vi "CAN 6 SPARK MAX Drivetrain Config.vi"() -> (14 "SPARK MAX Ref":T1={"FrontLeftMaster"={"DeviceStatus"={"status"=FALSE, "code"=0, "source"=""}, "Type"=enum."PWM", "PWM"={"PWM Channel"=enum."PWM 1", "DeadBand"={"Name"="", "maxPositivePwm"=0, "minPositivePwm"=0, "centerPwm"=0, "maxNegativePwm"=0, "minNegativePwm"=0, "angularRange"=0}}, "CAN"={"Device Number"=0, "SetOutput VI Ref"=variant(enum8{"Percent VBus", "Current", "Speed", "Position", "Voltage"} enum."Percent VBus"), "GetOutput VI Ref"=variant(refnum<k1> refnum), "Enable VI Ref"=variant(dbl 12.0), "Disable VI Ref"=variant(enum8{"Percent VBus", "Speed", "Position", "Slave", "Unchanged / Invalid", "Voltage Compensation", "Current", "Motion Profile"} enum."Percent VBus"), "Data"=variant}, "Invert"=FALSE, "DIO PWM"={"PWM \"Enable\" Channel"=enum."Invalid", "DIOChannel"=enum."Invalid", "PWM Rate"=0.0}}, "FrontLeftSlave1"={"DeviceStatus"={"status"=FALSE, "code"=0, "source"=""}, "Type"=enum."PWM", "PWM"={"PWM Channel"=enum."PWM 1", "DeadBand"={"Name"="", "maxPositivePwm"=0, "minPositivePwm"=0, "centerPwm"=0, "maxNegativePwm"=0, "minNegativePwm"=0, "angularRange"=0}}, "CAN"={"Device Number"=0, "SetOutput VI Ref"=variant(enum8{"Percent VBus", "Current", "Speed", "Position", "Voltage"} enum."Percent VBus"), "GetOutput VI Ref"=variant(refnum<k1> refnum), "Enable VI Ref"=variant(dbl 12.0), "Disable VI Ref"=variant(enum8{"Percent VBus", "Speed", "Position", "Slave", "Unchanged / Invalid", "Voltage Compensation", "Current", "Motion Profile"} enum."Percent VBus"), "Data"=variant}, "Invert"=FALSE, "DIO PWM"={"PWM \"Enable\" Channel"=enum."Invalid", "DIOChannel"=enum."Invalid", "PWM Rate"=0.0}}, "FrontLeftSlave2"={"DeviceStatus"={"status"=FALSE, "code"=0, "source"=""}, "Type"=enum."PWM", "PWM"={"PWM Channel"=enum."PWM 1", "DeadBand"={"Name"="", "maxPositivePwm"=0, "minPositivePwm"=0, "centerPwm"=0, "maxNegativePwm"=0, "minNegativePwm"=0, "angularRange"=0}}, "CAN"={"Device Number"=0, "SetOutput VI Ref"=variant(enum8{"Percent VBus", "Current", "Speed", "Position", "Voltage"} enum."Percent VBus"), "GetOutput VI Ref"=variant(refnum<k1> refnum), "Enable VI Ref"=variant(dbl 12.0), "Disable VI Ref"=variant(enum8{"Percent VBus", "Speed", "Position", "Slave", "Unchanged / Invalid", "Voltage Compensation", "Current", "Motion Profile"} enum."Percent VBus"), "Data"=variant}, "Invert"=FALSE, "DIO PWM"={"PWM \"Enable\" Channel"=enum."Invalid", "DIOChannel"=enum."Invalid", "PWM Rate"=0.0}}, "FrontRightMaster"={"DeviceStatus"={"status"=FALSE, "code"=0, "source"=""}, "Type"=enum."PWM", "PWM"={"PWM Channel"=enum."PWM 1", "DeadBand"={"Name"="", "maxPositivePwm"=0, "minPositivePwm"=0, "centerPwm"=0, "maxNegativePwm"=0, "minNegativePwm"=0, "angularRange"=0}}, "CAN"={"Device Number"=0, "SetOutput VI Ref"=variant(enum8{"Percent VBus", "Current", "Speed", "Position", "Voltage"} enum."Percent VBus"), "GetOutput VI Ref"=variant(refnum<k1> refnum), "Enable VI Ref"=variant(dbl 12.0), "Disable VI Ref"=variant(enum8{"Percent VBus", "Speed", "Position", "Slave", "Unchanged / Invalid", "Voltage Compensation", "Current", "Motion Profile"} enum."Percent VBus"), "Data"=variant}, "Invert"=FALSE, "DIO PWM"={"PWM \"Enable\" Channel"=enum."Invalid", "DIOChannel"=enum."Invalid", "PWM Rate"=0.0}}, "FrontRightSlave1"={"DeviceStatus"={"status"=FALSE, "code"=0, "source"=""}, "Type"=enum."PWM", "PWM"={"PWM Channel"=enum."PWM 1", "DeadBand"={"Name"="", "maxPositivePwm"=0, "minPositivePwm"=0, "centerPwm"=0, "maxNegativePwm"=0, "minNegativePwm"=0, "angularRange"=0}}, "CAN"={"Device Number"=0, "SetOutput VI Ref"=variant(enum8{"Percent VBus", "Current", "Speed", "Position", "Voltage"} enum."Percent VBus"), "GetOutput VI Ref"=variant(refnum<k1> refnum), "Enable VI Ref"=variant(dbl 12.0), "Disable VI Ref"=variant(enum8{"Percent VBus", "Speed", "Position", "Slave", "Unchanged / Invalid", "Voltage Compensation", "Current", "Motion Profile"} enum."Percent VBus"), "Data"=variant}, "Invert"=FALSE, "DIO PWM"={"PWM \"Enable\" Channel"=enum."Invalid", "DIOChannel"=enum."Invalid", "PWM Rate"=0.0}}, "FrontRightSlave2"={"DeviceStatus"={"status"=FALSE, "code"=0, "source"=""}, "Type"=enum."PWM", "PWM"={"PWM Channel"=enum."PWM 1", "DeadBand"={"Name"="", "maxPositivePwm"=0, "minPositivePwm"=0, "centerPwm"=0, "maxNegativePwm"=0, "minNegativePwm"=0, "angularRange"=0}}, "CAN"={"Device Number"=0, "SetOutput VI Ref"=variant(enum8{"Percent VBus", "Current", "Speed", "Position", "Voltage"} enum."Percent VBus"), "GetOutput VI Ref"=variant(refnum<k1> refnum), "Enable VI Ref"=variant(dbl 12.0), "Disable VI Ref"=variant(enum8{"Percent VBus", "Speed", "Position", "Slave", "Unchanged / Invalid", "Voltage Compensation", "Current", "Motion Profile"} enum."Percent VBus"), "Data"=variant}, "Invert"=FALSE, "DIO PWM"={"PWM \"Enable\" Channel"=enum."Invalid", "DIOChannel"=enum."Invalid", "PWM Rate"=0.0}}})   [LabVIEW 2018]
uses:
  SPARKMAX6Motor.ctl
  <vilib>/Rock Robotics/WPI/MotorControl/WPI_MotorControlDeviceRef.ctl
  <vilib>/Rock Robotics/WPI/MotorControl/WPI_MotorControlType.ctl
  <vilib>/Rock Robotics/SystemInterfaces/DIO/FPGA_DIOPWMChannel.ctl
  <vilib>/Rock Robotics/WPI/PWM/WPI_PWMDeadband.ctl
  <vilib>/Rock Robotics/SystemInterfaces/DIO/FPGA_DIOChannel.ctl
  <vilib>/Rock Robotics/WPI/ThirdParty/REV Robotics/SPARK MAX/Typedef/Spark MAX Status Frames.ctl
  <vilib>/Rock Robotics/WPI/ThirdParty/REV Robotics/SPARK MAX/Typedef/Spark MAX Idle Mode.ctl
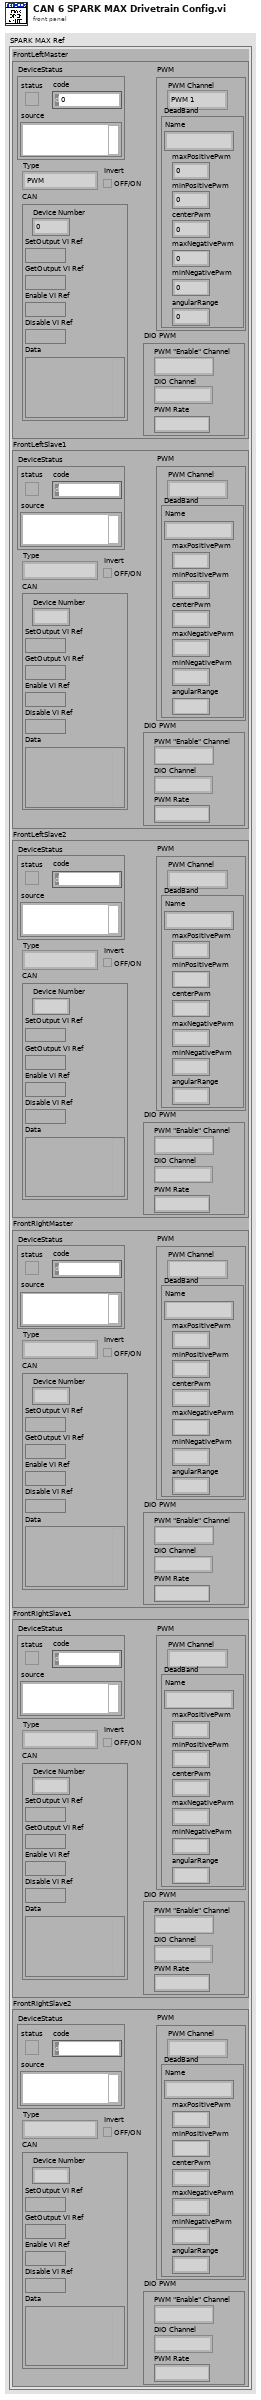
[diagram p1: front panel]
types:
  T1 = typedef "SPARKMAX6Motor.ctl" = cluster{"FrontLeftMaster":T2, "FrontLeftSlave1":T2, "FrontLeftSlave2":T2, "FrontRightMaster":T2, "FrontRightSlave1":T2, "FrontRightSlave2":T2}
  T2 = typedef "WPI_MotorControlDeviceRef.ctl" = cluster{"DeviceStatus":errorcluster, "Type":T3, "PWM":cluster{"PWM Channel":T4, "DeadBand":T5}, "CAN":cluster{"Device Number":u8, "SetOutput VI Ref":variant, "GetOutput VI Ref":variant, "Enable VI Ref":variant, "Disable VI Ref":variant, "Data":variant}, "Invert":bool, "DIO PWM":cluster{"PWM \"Enable\" Channel":T4, "DIOChannel":T6, "PWM Rate":dbl}}
  T3 = typedef "WPI_MotorControlType.ctl" = enum16{"PWM", "CAN", "DIO PWM"}
  T4 = typedef "FPGA_DIOPWMChannel.ctl" = enum8{"PWM 0", "PWM 1", "PWM 2", "PWM 3", "PWM 4", "PWM 5", "PWM 6", "PWM 7", "PWM 8", "PWM 9", "PWM MXP 0", "PWM MXP 1", "PWM MXP 2", "PWM MXP 3", "PWM MXP 4", "PWM MXP 5", "PWM MXP 6", "PWM MXP 7", "PWM MXP 8", "PWM MXP 9", "Invalid"}
  T5 = typedef "WPI_PWMDeadband.ctl" = cluster{"Name":string, "maxPositivePwm":i32, "minPositivePwm":i32, "centerPwm":i32, "maxNegativePwm":i32, "minNegativePwm":i32, "angularRange":u16}
  T6 = typedef "FPGA_DIOChannel.ctl" = enum8{"DIO 0", "DIO 1", "DIO 2", "DIO 3", "DIO 4", "DIO 5", "DIO 6", "DIO 7", "DIO 8", "DIO 9", "DIO MXP 0", "DIO MXP 1", "DIO MXP 2", "DIO MXP 3", "DIO MXP 4", "DIO MXP 5", "DIO MXP 6", "DIO MXP 7", "DIO MXP 8", "DIO MXP 9", "DIO MXP 10", "DIO MXP 11", "DIO MXP 12", "DIO MXP 13", "DIO MXP 14", "DIO MXP 15", "SPI Port CS1", "SPI Port CS2", "SPI Port CS3", "SPI Port MISO", "SPI Port MOSI", "Invalid"}
  T7 = typedef "Spark MAX Idle Mode.ctl" = enum16{"Coast", "Brake"}
  T8 = typedef "Spark MAX Status Frames.ctl" = enum16{"Status 0", "Status 1", "Status 2"}
  T9 = cluster{"P Gain":dbl, "I Gain":dbl, "D Gain":dbl, "F Gain":dbl, "I Zone":dbl, "Min Output":dbl, "Max Output":dbl}
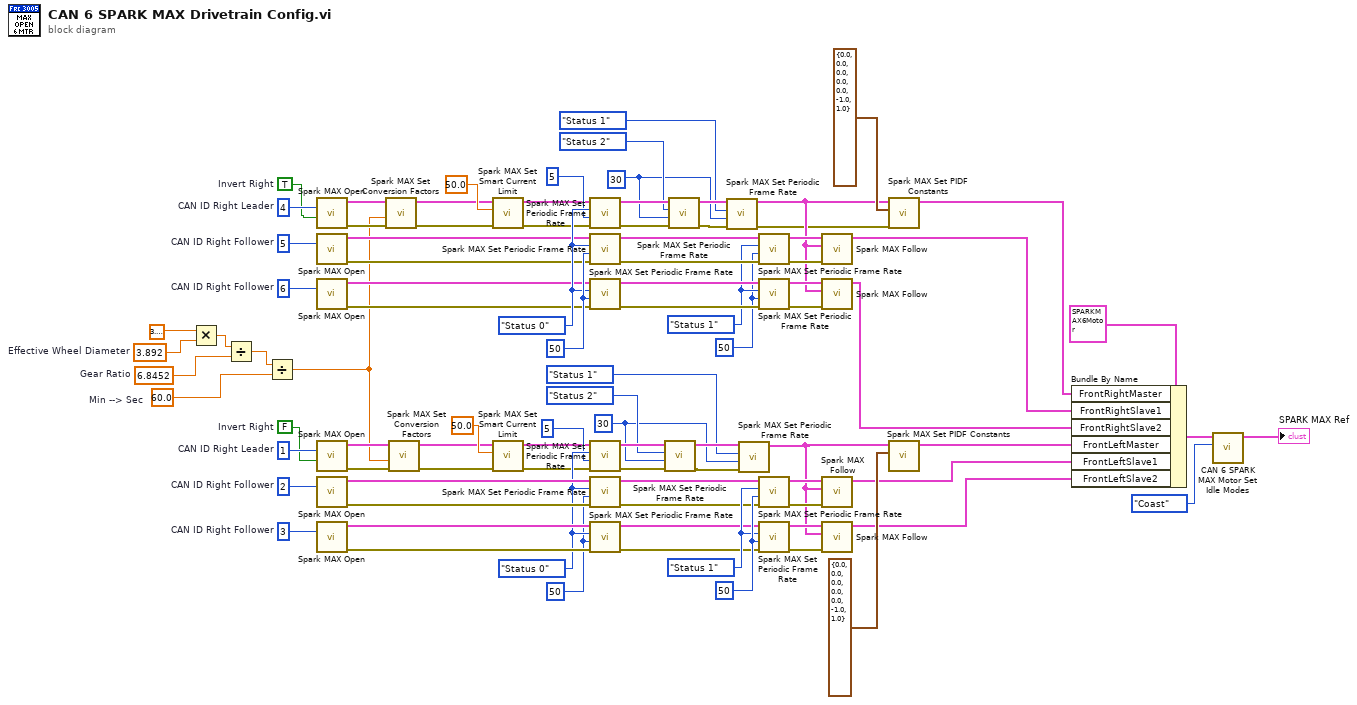
[diagram p0: block diagram]
diagram:
  w1 = 3.892  # Effective Wheel Diameter
  w2 = 6.8452  # Gear Ratio
  w3 = 60.0  # Min --> Sec
  w61 = u16 50 ("Frame rate (ms)")
  w62 = Spark_MAX_Status_Frames."Status 1" ("Frame")
  w60 = u16 50 ("Frame rate (ms)")
  w26 = u16 30 ("Frame rate (ms)")
  w59 = Spark_MAX_Status_Frames."Status 0" ("Frame")
  w54 = u8 6  # CAN ID Right Follower
  w28 = TRUE  # Invert Right
  w52 = u8 4  # CAN ID Right Leader
  w53 = u8 5  # CAN ID Right Follower
  w82 = u16 50 ("Frame rate (ms)")
  w81 = Spark_MAX_Status_Frames."Status 1" ("Frame")
  w83 = u16 50 ("Frame rate (ms)")
  w29 = u16 30 ("Frame rate (ms)")
  w84 = Spark_MAX_Status_Frames."Status 0" ("Frame")
  w90 = u8 3  # CAN ID Right Follower
  w27 = FALSE  # Invert Right
  w92 = u8 1  # CAN ID Right Leader
  w91 = u8 2  # CAN ID Right Follower
  n1 = Multiply(x=3.141592653589793, y=w1) -> (x*y=w5:dbl)
  n2 = Divide(x=w5, y=w2) -> (x/y=w6:dbl)
  n3 = Divide(x=w6, y=w3) -> (x/y=w4:dbl)
  n4 = call <vilib>:"Spark MAX Open.vi"("Invert"=w28, "Device Number"=w52) -> ("error out"=w14:errorcluster, "MotorControlDeviceRef"=w12:T2)  [unwired: 8 in]
  n5 = call <vilib>:"Spark MAX Open.vi"("Device Number"=w53) -> ("error out"=w57:errorcluster, "MotorControlDeviceRef"=w58:T2)  [unwired: 9 in]
  n6 = call <vilib>:"Spark MAX Open.vi"("Device Number"=w54) -> ("error out"=w55:errorcluster, "MotorControlDeviceRef"=w56:T2)  [unwired: 9 in]
  n7 = call <vilib>:"Spark MAX Open.vi"("Invert"=w27, "Device Number"=w92) -> ("error out"=w85:errorcluster, "MotorControlDeviceRef"=w9:T2)  [unwired: 8 in]
  n8 = call <vilib>:"Spark MAX Open.vi"("Device Number"=w91) -> ("error out"=w87:errorcluster, "MotorControlDeviceRef"=w86:T2)  [unwired: 9 in]
  n9 = call <vilib>:"Spark MAX Open.vi"("Device Number"=w90) -> ("error out"=w89:errorcluster, "MotorControlDeviceRef"=w88:T2)  [unwired: 9 in]
  n10 = call <vilib>:"Spark MAX Set Conversion Factors.vi"("error in (no error)"=w14, "Velocity Factor (1)"=w4, "MotorControlDeviceRef in"=w12) -> ("error out"=w13:errorcluster, "MotorControlDeviceRef out"=w11:T2)  [unwired: 7 in]
  n11 = call <vilib>:"Spark MAX Set Conversion Factors.vi"("error in (no error)"=w85, "Velocity Factor (1)"=w4, "MotorControlDeviceRef in"=w9) -> ("error out"=w10:errorcluster, "MotorControlDeviceRef out"=w8:T2)  [unwired: 7 in]
  n12 = call <vilib>:"Spark MAX Set Smart Current Limit.vi"("error in (no error)"=w13, "Primay Current Limit (80A)"=50.0, "MotorControlDeviceRef in"=w11) -> ("error out"=w20:errorcluster, "MotorControlDeviceRef out"=w19:T2)  [unwired: 7 in]
  n13 = call <vilib>:"Spark MAX Set Smart Current Limit.vi"("error in (no error)"=w10, "Primay Current Limit (80A)"=50.0, "MotorControlDeviceRef in"=w8) -> ("error out"=w18:errorcluster, "MotorControlDeviceRef out"=w17:T2)  [unwired: 7 in]
  n14 = call <vilib>:"Spark MAX Set Periodic Frame Rate.vi"("error in"=w20, "Frame rate (ms)"=u16 5, "Frame"=w59, "MotorControlDeviceRef"=w19) -> ("error out"=w44:errorcluster, "MotorControlDeviceRef"=w43:T2)  [unwired: 6 in]
  n15 = call <vilib>:"Spark MAX Set Periodic Frame Rate.vi"("error in"=w57, "Frame rate (ms)"=w60, "Frame"=w59, "MotorControlDeviceRef"=w58) -> ("error out"=w66:errorcluster, "MotorControlDeviceRef"=w63:T2)  [unwired: 6 in]
  n16 = call <vilib>:"Spark MAX Set Periodic Frame Rate.vi"("error in"=w55, "Frame rate (ms)"=w60, "Frame"=w59, "MotorControlDeviceRef"=w56) -> ("error out"=w65:errorcluster, "MotorControlDeviceRef"=w64:T2)  [unwired: 6 in]
  n17 = call <vilib>:"Spark MAX Set Periodic Frame Rate.vi"("error in"=w18, "Frame rate (ms)"=u16 5, "Frame"=w84, "MotorControlDeviceRef"=w17) -> ("error out"=w33:errorcluster, "MotorControlDeviceRef"=w34:T2)  [unwired: 6 in]
  n18 = call <vilib>:"Spark MAX Set Periodic Frame Rate.vi"("error in"=w87, "Frame rate (ms)"=w83, "Frame"=w84, "MotorControlDeviceRef"=w86) -> ("error out"=w77:errorcluster, "MotorControlDeviceRef"=w80:T2)  [unwired: 6 in]
  n19 = call <vilib>:"Spark MAX Set Periodic Frame Rate.vi"("error in"=w89, "Frame rate (ms)"=w83, "Frame"=w84, "MotorControlDeviceRef"=w88) -> ("error out"=w78:errorcluster, "MotorControlDeviceRef"=w79:T2)  [unwired: 6 in]
  n20 = call <vilib>:"Spark MAX Set Periodic Frame Rate.vi"("error in"=w33, "Frame rate (ms)"=w29, "Frame"=Spark_MAX_Status_Frames."Status 2", "MotorControlDeviceRef"=w34) -> ("error out"=w36:errorcluster, "MotorControlDeviceRef"=w35:T2)  [unwired: 6 in]
  n21 = call <vilib>:"Spark MAX Set Periodic Frame Rate.vi"("error in"=w44, "Frame rate (ms)"=w26, "Frame"=Spark_MAX_Status_Frames."Status 2", "MotorControlDeviceRef"=w43) -> ("error out"=w41:errorcluster, "MotorControlDeviceRef"=w42:T2)  [unwired: 6 in]
  n22 = call <vilib>:"Spark MAX Set Periodic Frame Rate.vi"("error in"=w41, "Frame rate (ms)"=w26, "Frame"=Spark_MAX_Status_Frames."Status 1", "MotorControlDeviceRef"=w42) -> ("error out"=w37:errorcluster, "MotorControlDeviceRef"=w38:T2)  [unwired: 6 in]
  n23 = call <vilib>:"Spark MAX Set Periodic Frame Rate.vi"("error in"=w36, "Frame rate (ms)"=w29, "Frame"=Spark_MAX_Status_Frames."Status 1", "MotorControlDeviceRef"=w35) -> ("MotorControlDeviceRef"=w32:T2)  [unwired: 6 in, 1 out]
  n24 = call <vilib>:"Spark MAX Set Periodic Frame Rate.vi"("error in"=w66, "Frame rate (ms)"=w61, "Frame"=w62, "MotorControlDeviceRef"=w63) -> ("error out"=w68:errorcluster, "MotorControlDeviceRef"=w67:T2)  [unwired: 6 in]
  n25 = call <vilib>:"Spark MAX Set Periodic Frame Rate.vi"("error in"=w65, "Frame rate (ms)"=w61, "Frame"=w62, "MotorControlDeviceRef"=w64) -> ("error out"=w69:errorcluster, "MotorControlDeviceRef"=w70:T2)  [unwired: 6 in]
  n26 = call <vilib>:"Spark MAX Set Periodic Frame Rate.vi"("error in"=w77, "Frame rate (ms)"=w82, "Frame"=w81, "MotorControlDeviceRef"=w80) -> ("error out"=w75:errorcluster, "MotorControlDeviceRef"=w76:T2)  [unwired: 6 in]
  n27 = call <vilib>:"Spark MAX Set Periodic Frame Rate.vi"("error in"=w78, "Frame rate (ms)"=w82, "Frame"=w81, "MotorControlDeviceRef"=w79) -> ("error out"=w74:errorcluster, "MotorControlDeviceRef"=w73:T2)  [unwired: 6 in]
  n28 = call <vilib>:"Spark MAX Follow.vi"("error in (no error)"=w68, "Master Controller"=w38, "MotorControlDeviceRef"=w67) -> ("MotorControlDeviceRef"=w45:T2)  [unwired: 7 in, 1 out]
  n29 = call <vilib>:"Spark MAX Follow.vi"("error in (no error)"=w69, "Master Controller"=w38, "MotorControlDeviceRef"=w70) -> ("MotorControlDeviceRef"=w46:T2)  [unwired: 7 in, 1 out]
  n30 = call <vilib>:"Spark MAX Follow.vi"("error in (no error)"=w75, "Master Controller"=w32, "MotorControlDeviceRef"=w76) -> ("MotorControlDeviceRef"=w48:T2)  [unwired: 7 in, 1 out]
  n31 = call <vilib>:"Spark MAX Follow.vi"("error in (no error)"=w74, "Master Controller"=w32, "MotorControlDeviceRef"=w73) -> ("MotorControlDeviceRef"=w47:T2)  [unwired: 7 in, 1 out]
  n32 = call <vilib>:"Spark MAX Set PIDF Constants.vi"("error in"=w37, "PID Constants"=T9 {"P Gain"=0.0, "I Gain"=0.0, "D Gain"=0.0, "F Gain"=0.0, "I Zone"=0.0, "Min Output"=-1.0, "Max Output"=1.0}, "MotorControlDeviceRef"=w38) -> ("MotorControlDeviceRef"=w50:T2)  [unwired: 7 in, 1 out]
  n33 = call <vilib>:"Spark MAX Set PIDF Constants.vi"("PID Constants"=T9 {"P Gain"=0.0, "I Gain"=0.0, "D Gain"=0.0, "F Gain"=0.0, "I Zone"=0.0, "Min Output"=-1.0, "Max Output"=1.0}, "MotorControlDeviceRef"=w32) -> ("MotorControlDeviceRef"=w49:T2)  [unwired: 8 in, 1 out]
  n34 = Bundle By Name(cluster=T1 {"FrontLeftMaster"={"DeviceStatus"={"status"=FALSE, "code"=0, "source"=""}, "Type"=enum."PWM", "PWM"={"PWM Channel"=enum."PWM 1", "DeadBand"={"Name"="", "maxPositivePwm"=0, "minPositivePwm"=0, "centerPwm"=0, "maxNegativePwm"=0, "minNegativePwm"=0, "angularRange"=0}}, "CAN"={"Device Number"=0, "SetOutput VI Ref"=variant(enum8{"Percent VBus", "Current", "Speed", "Position", "Voltage"} enum."Percent VBus"), "GetOutput VI Ref"=variant(refnum<k1> refnum), "Enable VI Ref"=variant(dbl 12.0), "Disable VI Ref"=variant(enum8{"Percent VBus", "Speed", "Position", "Slave", "Unchanged / Invalid", "Voltage Compensation", "Current", "Motion Profile"} enum."Percent VBus"), "Data"=variant}, "Invert"=FALSE, "DIO PWM"={"PWM \"Enable\" Channel"=enum."Invalid", "DIOChannel"=enum."Invalid", "PWM Rate"=0.0}}, "FrontLeftSlave1"={"DeviceStatus"={"status"=FALSE, "code"=0, "source"=""}, "Type"=enum."PWM", "PWM"={"PWM Channel"=enum."PWM 1", "DeadBand"={"Name"="", "maxPositivePwm"=0, "minPositivePwm"=0, "centerPwm"=0, "maxNegativePwm"=0, "minNegativePwm"=0, "angularRange"=0}}, "CAN"={"Device Number"=0, "SetOutput VI Ref"=variant(enum8{"Percent VBus", "Current", "Speed", "Position", "Voltage"} enum."Percent VBus"), "GetOutput VI Ref"=variant(refnum<k1> refnum), "Enable VI Ref"=variant(dbl 12.0), "Disable VI Ref"=variant(enum8{"Percent VBus", "Speed", "Position", "Slave", "Unchanged / Invalid", "Voltage Compensation", "Current", "Motion Profile"} enum."Percent VBus"), "Data"=variant}, "Invert"=FALSE, "DIO PWM"={"PWM \"Enable\" Channel"=enum."Invalid", "DIOChannel"=enum."Invalid", "PWM Rate"=0.0}}, "FrontLeftSlave2"={"DeviceStatus"={"status"=FALSE, "code"=0, "source"=""}, "Type"=enum."PWM", "PWM"={"PWM Channel"=enum."PWM 1", "DeadBand"={"Name"="", "maxPositivePwm"=0, "minPositivePwm"=0, "centerPwm"=0, "maxNegativePwm"=0, "minNegativePwm"=0, "angularRange"=0}}, "CAN"={"Device Number"=0, "SetOutput VI Ref"=variant(enum8{"Percent VBus", "Current", "Speed", "Position", "Voltage"} enum."Percent VBus"), "GetOutput VI Ref"=variant(refnum<k1> refnum), "Enable VI Ref"=variant(dbl 12.0), "Disable VI Ref"=variant(enum8{"Percent VBus", "Speed", "Position", "Slave", "Unchanged / Invalid", "Voltage Compensation", "Current", "Motion Profile"} enum."Percent VBus"), "Data"=variant}, "Invert"=FALSE, "DIO PWM"={"PWM \"Enable\" Channel"=enum."Invalid", "DIOChannel"=enum."Invalid", "PWM Rate"=0.0}}, "FrontRightMaster"={"DeviceStatus"={"status"=FALSE, "code"=0, "source"=""}, "Type"=enum."PWM", "PWM"={"PWM Channel"=enum."PWM 1", "DeadBand"={"Name"="", "maxPositivePwm"=0, "minPositivePwm"=0, "centerPwm"=0, "maxNegativePwm"=0, "minNegativePwm"=0, "angularRange"=0}}, "CAN"={"Device Number"=0, "SetOutput VI Ref"=variant(enum8{"Percent VBus", "Current", "Speed", "Position", "Voltage"} enum."Percent VBus"), "GetOutput VI Ref"=variant(refnum<k1> refnum), "Enable VI Ref"=variant(dbl 12.0), "Disable VI Ref"=variant(enum8{"Percent VBus", "Speed", "Position", "Slave", "Unchanged / Invalid", "Voltage Compensation", "Current", "Motion Profile"} enum."Percent VBus"), "Data"=variant}, "Invert"=FALSE, "DIO PWM"={"PWM \"Enable\" Channel"=enum."Invalid", "DIOChannel"=enum."Invalid", "PWM Rate"=0.0}}, "FrontRightSlave1"={"DeviceStatus"={"status"=FALSE, "code"=0, "source"=""}, "Type"=enum."PWM", "PWM"={"PWM Channel"=enum."PWM 1", "DeadBand"={"Name"="", "maxPositivePwm"=0, "minPositivePwm"=0, "centerPwm"=0, "maxNegativePwm"=0, "minNegativePwm"=0, "angularRange"=0}}, "CAN"={"Device Number"=0, "SetOutput VI Ref"=variant(enum8{"Percent VBus", "Current", "Speed", "Position", "Voltage"} enum."Percent VBus"), "GetOutput VI Ref"=variant(refnum<k1> refnum), "Enable VI Ref"=variant(dbl 12.0), "Disable VI Ref"=variant(enum8{"Percent VBus", "Speed", "Position", "Slave", "Unchanged / Invalid", "Voltage Compensation", "Current", "Motion Profile"} enum."Percent VBus"), "Data"=variant}, "Invert"=FALSE, "DIO PWM"={"PWM \"Enable\" Channel"=enum."Invalid", "DIOChannel"=enum."Invalid", "PWM Rate"=0.0}}, "FrontRightSlave2"={"DeviceStatus"={"status"=FALSE, "code"=0, "source"=""}, "Type"=enum."PWM", "PWM"={"PWM Channel"=enum."PWM 1", "DeadBand"={"Name"="", "maxPositivePwm"=0, "minPositivePwm"=0, "centerPwm"=0, "maxNegativePwm"=0, "minNegativePwm"=0, "angularRange"=0}}, "CAN"={"Device Number"=0, "SetOutput VI Ref"=variant(enum8{"Percent VBus", "Current", "Speed", "Position", "Voltage"} enum."Percent VBus"), "GetOutput VI Ref"=variant(refnum<k1> refnum), "Enable VI Ref"=variant(dbl 12.0), "Disable VI Ref"=variant(enum8{"Percent VBus", "Speed", "Position", "Slave", "Unchanged / Invalid", "Voltage Compensation", "Current", "Motion Profile"} enum."Percent VBus"), "Data"=variant}, "Invert"=FALSE, "DIO PWM"={"PWM \"Enable\" Channel"=enum."Invalid", "DIOChannel"=enum."Invalid", "PWM Rate"=0.0}}} ("TalonSRX6Motor"), "FrontRightMaster"=w50, "FrontRightSlave1"=w45, "FrontRightSlave2"=w46, "FrontLeftMaster"=w49, "FrontLeftSlave1"=w48, "FrontLeftSlave2"=w47) -> (w23:T1)
  n35 = call "CAN 6 SPARK MAX Motor Set Idle Modes.vi"("Idle Mode"=Spark_MAX_Idle_Mode."Coast", "SPARK MAX ref in"=w23) -> ("SPARK MAX ref"=→"SPARK MAX Ref":T1)  [unwired: 8 in, 1 out]
